vi "Read Channel Index.vi"(8 "error in (no error)":errorcluster, 11 "Digital Toggle Single Msg in":refnum<class "Digital Toggle Single Msg.lvclass">) -> (0 "error out":errorcluster, 2 "Channel Index":i32, 3 "Digital Toggle Single Msg out":refnum<class "Digital Toggle Single Msg.lvclass">)   [LabVIEW 2024, in "DAQmx Actor.lvlib" / "Digital Toggle Single Msg.lvclass"]
uses:
  Digital Toggle Single Msg.lvclass
  Digital Toggle Single Msg.lvclass/Digital Toggle Single Msg.ctl
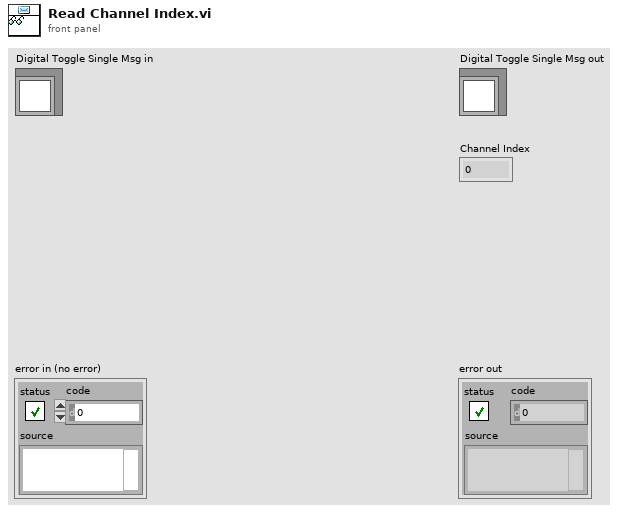
[diagram p1: front panel]
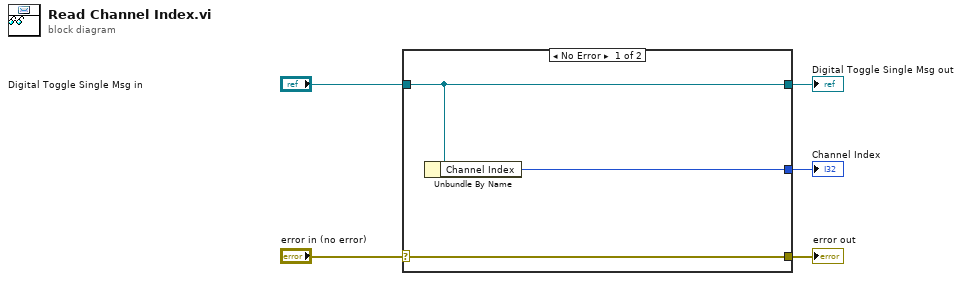
[diagram p0: block diagram]
diagram:
  n1 = case shown="No Error" "error in (no error)" {
    selector: "error in (no error)" -> [w8 w9]
    tunnel: [w8 w9] -> w4
    tunnel: [w7 w10] -> w2
    tunnel: "Digital Toggle Single Msg in" -> [w7 w10]
    tunnel: [w6 _] -> w1
    frame No Error {
      n2 = Unbundle By Name(w7) -> ("Channel Index"=w6:i32)
    }
    frame Error {
    }
  }
  "error out" <- w4
  "Digital Toggle Single Msg out" <- w2
  "Channel Index" <- w1
